vi "VoltageScan_datastream.vi"() -> ()   [LabVIEW 2015]
uses:
  Dynamic_data.ctl
  Program Files (x86)/National Instruments/LabVIEW 2016/instr.lib/Keithley 24XX/Keithley 24XX.lvlib
  Program Files (x86)/National Instruments/LabVIEW 2016/instr.lib/Agilent 428X Series/Agilent 428X Series.lvlib
  Program Files (x86)/National Instruments/LabVIEW 2016/instr.lib/Keithley 24XX/Public/Data/Read (Single Point).vi
  Input_parameters.ctl
panel:
  out "Voltages":cluster{"X":dbl[], "Y":dbl[]}[](graph) caption="XY Graph"
  out "Current channel":i32
  out "Channels":cluster{i32[], dbl[]}[](graph) caption="XY Graph"
  in  "Stop":bool
  out "Current voltage [V]":dbl
  out "Data curve for single channel":cluster{"X":dbl[], "Y":dbl[]}[](graph) caption="XY Graph"
  in  "Input parameters":T1={"Measurement type"=enum."Test", "Sensor type"=enum."One channel", "Input file"="", "Output file"="test.txt", "Open after execution?"=FALSE, "Display channel"=0, "Voltage Delay (s)"=0.5, "Switch Delay (s)"=0.01, "VISA resource name source"="", "VISA resource name LCR"="", "Voltage Limit (V)"=1000.0, "Enable Voltage Auto Range (T:Enable)"=TRUE, "Voltage Manual Range (1.0)"=1.0, "Compliance  Level (uA)"=10.0} {"Voltage Limit (V)" format="%#_13g"; "Voltage Delay (s)" format="%#_13g"; "Switch Delay (s)" format="%#_13g"}
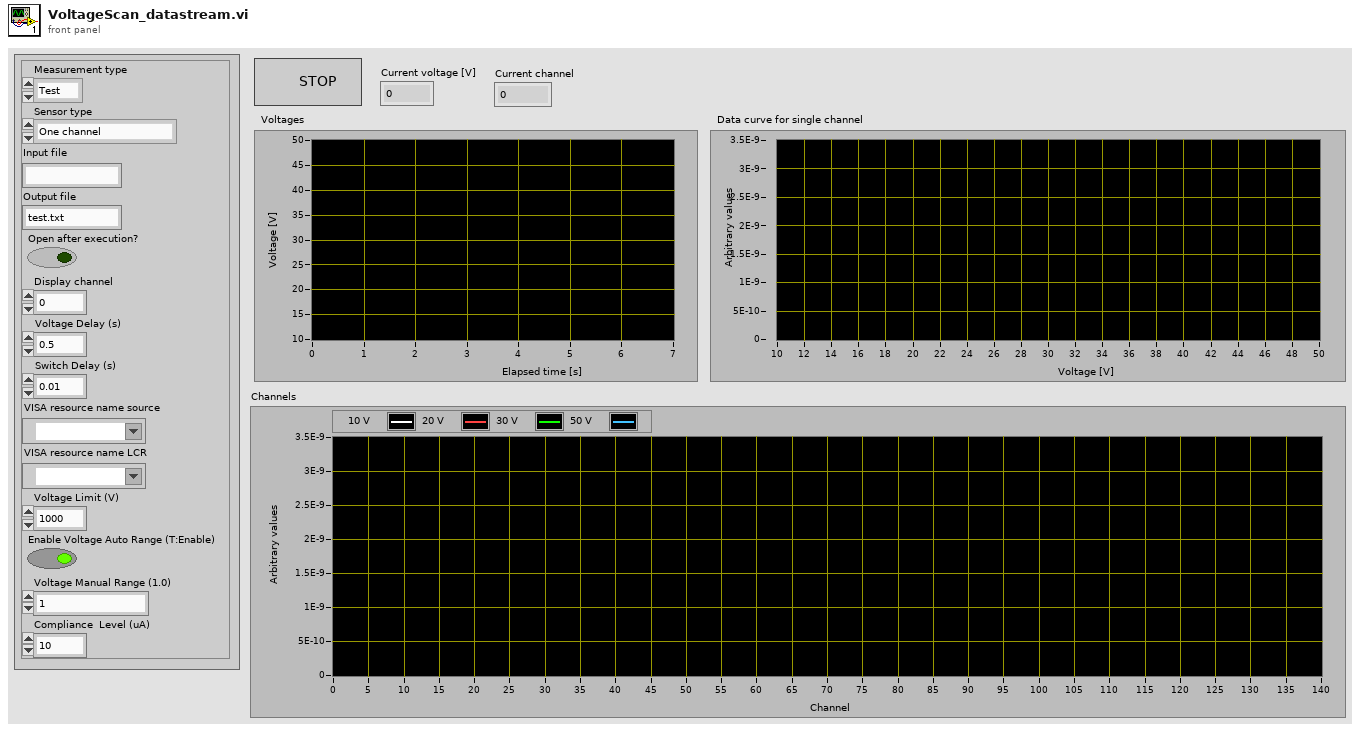
[diagram p1: front panel]
types:
  T1 = typedef "Input_parameters.ctl" = cluster{"Measurement type":enum16{"IV", "CV", "Test"}, "Sensor type":enum16{"6''", "8''", "One channel"}, "Input file":string, "Output file":string, "Open after execution?":bool, "Display channel":i32, "Voltage Delay (s)":dbl, "Switch Delay (s)":dbl, "VISA resource name source":refnum<visa-resource-name>, "VISA resource name LCR":refnum<visa-resource-name>, "Voltage Limit (V)":dbl, "Enable Voltage Auto Range (T:Enable)":bool, "Voltage Manual Range (1.0)":dbl, "Compliance  Level (uA)":dbl}
  T2 = typedef "Dynamic_data.ctl" = cluster{"Input file":path, "Output file":path, "Y-label text":string, "Voltage array":dbl[][], "Current set voltage":dbl, "Voltage column":dbl[], "Pad number column":dbl[], "Data  column":dbl[], "Number of voltages":i32, "Compliance current (A)":dbl}
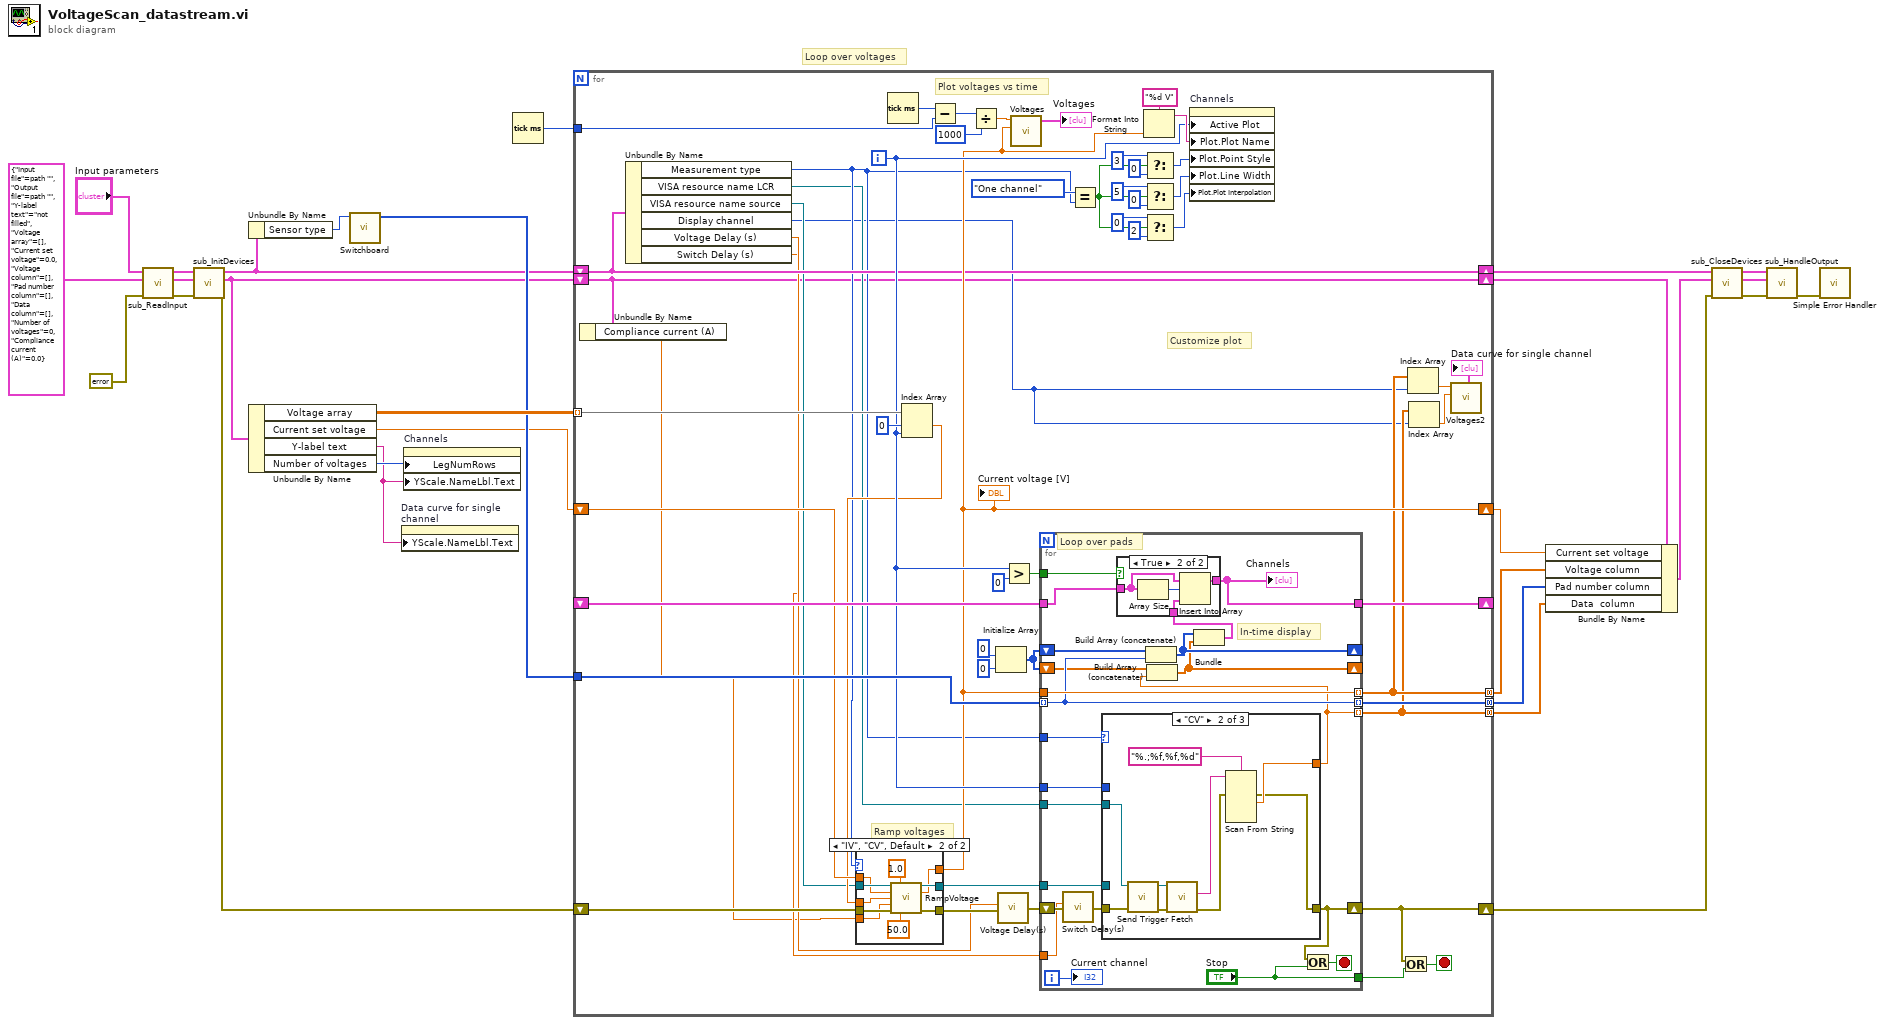
[diagram p0: block diagram]
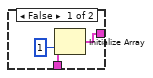
[diagram p3: hidden frame]
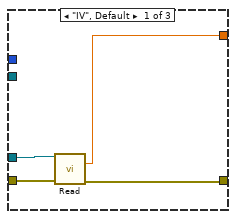
[diagram p4: hidden frame]
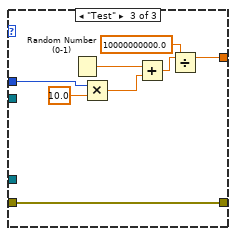
[diagram p5: hidden frame]
diagram:
  # "Loop over voltages"
  n1 = call "sub_ReadInput.vi"("error in (no error)"=errorcluster {"status"=FALSE, "code"=0, "source"=""}, "Dynamic data"=T2 {"Input file"=path "", "Output file"=path "", "Y-label text"="not filled", "Voltage array"=[], "Current set voltage"=0.0, "Voltage column"=[], "Pad number column"=[], "Data  column"=[], "Number of voltages"=0, "Compliance current (A)"=0.0}, "Input parameters"="Input parameters") -> ("error out"=w25:errorcluster, "Dynamic data"=w20:T2, "Input parameters"=w26:T1)  [unwired: 6 in]
  n2 = call "sub_InitDevices.vi"("error in (no error)"=w25, "Dynamic data"=w20, "Input parameters"=w26) -> ("error out"=w13:errorcluster, "Dynamic data"=w3:T2, "Input parameters"=w4:T1)  [unwired: 6 in]
  n3 = Unbundle By Name(w4) -> ("Sensor type"=w18:enum16{"6''", "8''", "One channel"})
  n4 = Unbundle By Name(w3) -> ("Voltage array"=w17:dbl[][], "Current set voltage"=w14:dbl, "Y-label text"=w5:string, "Number of voltages"=w6:i32)
  n5 = call "Switchboard.vi"("Sensor type"=w18) -> ("Output config"=w15:i32[])  [unwired: 10 in]
  n6 = property on="Data curve for single channel" class="XYGraph (strict)"("YScale.NameLbl.Text"=w5) -> ()  [unwired: 2 in, 2 out]
  n7 = property on="Channels" class="XYGraph (strict)"("LegNumRows"=w6, "YScale.NameLbl.Text"=w5) -> ()  [unwired: 2 in, 2 out]
  n8 = Tick Count (ms)() -> (millisecond timer value=w16:u32)
  n9 = for {
    tunnel: w17 -> [w83] mode=indexing
    tunnel: w15 -> [w80]
    tunnel: [w44] -> w9 mode=concatenating
    tunnel: [w43] -> w7 mode=concatenating
    tunnel: [w78] -> w8 mode=concatenating
    shift-right: [w48] -> w12
    shift-left: w13 -> [w76]
    shift-right: [w72] -> _
    shift-left: _ -> [w71]
    tunnel: w16 -> [w65]
    shift-right: [w45] -> w10
    shift-left: w14 -> [w47]
    shift-right: [w38] -> w2
    shift-left: w4 -> [w38]
    shift-right: [w30] -> w1
    shift-left: w3 -> [w30]
    i -> [w51]
    stop <- w49 stop-if-true
    # "Ramp voltages"
    # "Plot voltages vs time"
    # "Customize plot"
    n10 = Unbundle By Name(w30) -> ("Compliance current (A)"=w29:dbl)
    n11 = Unbundle By Name(w38) -> ("Measurement type"=w36:enum16{"IV", "CV", "Test"}, "VISA resource name LCR"=w34:refnum<visa-resource-name>, "VISA resource name source"=w35:refnum<visa-resource-name>, "Display channel"=w33:i32, "Voltage Delay (s)"=w32:dbl, "Switch Delay (s)"=w31:dbl)
    n12 = Tick Count (ms)() -> (millisecond timer value=w67:u32)
    n13 = Index Array(array=w83, index #1=0 ("index"), index #2=w51) -> (element #1=w46:dbl)  [unwired: 1 out]
    n14 = case shown="\"IV\", \"CV\", Default" w36 {
      tunnel: w35 -> [w86 w93]
      tunnel: w46 -> [w84 w92]
      tunnel: [w86 w95] -> w77
      tunnel: w76 -> [w85 w94]
      tunnel: [w85 w96] -> w75
      tunnel: w29 -> [_ w90]
      tunnel: w47 -> [_ w91]
      tunnel: [w84 w87] -> w45
      frame "Test" {
      }
      frame "IV", "CV", Default {
        n15 = call "RampVoltage.vi"("VISA resource name"=w93, "Delay (s)"=1.0, "Current voltage (V)"=w91, "Target voltage (V)"=w92, "Compliance Current (A)"=w90, "error in (no error)"=w94, "Step size (V)"=50.0) -> ("VISA resource name out"=w95:refnum<visa-resource-name>, "Current voltage out (V)"=w87:dbl, "error out"=w96:errorcluster)  [unwired: 6 in]
      }
    }
    "Current voltage [V]" <- w45
    n16 = Subtract(x=w67, y=w65) -> (x-y=w66:u32)
    n17 = Divide(x=w66, y=u32 1000 ("x")) -> (x/y=w64:dbl)
    n18 = Initialize Array(0 ("dimension size"), 0 ("dimension size")) -> (w68:i32[])
    n19 = call "Voltage Delay(s)"("error in (no error)"=w75, "Delay Time (s)"=w32) -> ("error out"=w74:errorcluster)  [unwired: 9 in]
    n20 = Greater?(x=w51, y=0) -> (0:w73:bool)
    n21 = call "Voltages"("Y Input"=w45, "X Input"=w64) -> ("XY Graph"=→"Voltages":cluster{"X":dbl[], "Y":dbl[]}[])  [unwired: 8 in, 1 out]
    n22 = for {
      tunnel: w80 -> [w114] mode=indexing
      tunnel: [w114] -> w78 mode=indexing
      tunnel: [w112] -> w43 mode=indexing
      tunnel: w45 -> [w118]
      tunnel: [w118] -> w44 mode=indexing
      tunnel: w77 -> [w116]
      tunnel: w36 -> [w117]
      shift-right: [w100] -> w48
      shift-left: w74 -> [w101]
      tunnel: w34 -> [w115]
      shift-right: [w110] -> _
      shift-left: w68 -> [w113]
      shift-right: [w109] -> _
      shift-left: w68 -> [w111]
      tunnel: w73 -> [w107]
      tunnel: w51 -> [w108]
      tunnel: w71 -> [w106]
      tunnel: [w104] -> w72
      tunnel: ["Stop"] -> w50
      tunnel: w31 -> [w97]
      i -> [w105]
      stop <- w99 stop-if-true
      # "In-time display"
      # "Loop over pads"
      n23 = call "Switch Delay(s)"("error in (no error)"=w101, "Delay Time (s)"=w97) -> ("error out"=w102:errorcluster)  [unwired: 9 in]
      n24 = case shown="\"CV\"" w117 {
        tunnel: [w129 w132 w140] -> w112
        tunnel: w116 -> [w127 _ _]
        tunnel: w102 -> [w128 w135 w146]
        tunnel: [w126 w130 w146] -> w100
        tunnel: w115 -> [_ w136 _]
        tunnel: w108 -> [_ _ w141]
        frame "IV", Default {
          n25 = call-poly "Read.vi"("VISA resource name"=w127, "error in (no error)"=w128) -> ("Current"=w129:sgl, "error out"=w126:errorcluster)  [unwired: 7 in, 5 out]
        }
        frame "CV" {
          n26 = call "Send Trigger.vi"("error in (no error)"=w135, "VISA resource name"=w136) -> ("error out"=w137:errorcluster, "VISA resource name out"=w138:refnum<visa-resource-name>)  [unwired: 8 in]
          n27 = call "Fetch.vi"("error in (no error)"=w137, "VISA resource name"=w138) -> ("error out"=w131:errorcluster, "Returned Data"=w133:string)  [unwired: 7 in, 1 out]
          n28 = Scan From String(format string="%.;%f,%f,%d", input string=w133, error in=w131) -> (error out=w130:errorcluster, output 1=w132:dbl)  [unwired: 6 in, 2 out]
        }
        frame "Test" {
          n29 = Random Number (0-1)() -> (number: 0 to 1=w145:dbl)
          n30 = Multiply(x=w141, y=10.0) -> (x*y=w142:dbl)
          n31 = Add(x=w145, y=w142) -> (x+y=w144:dbl)
          n32 = Divide(x=w144, y=10000000000.0) -> (x/y=w140:dbl)
        }
      }
      n33 = Build Array (concatenate)(w113, w114) -> (w110:i32[])
      n34 = Build Array (concatenate)(w111, w112) -> (w109:dbl[])
      n35 = Bundle(w110, w109) -> (w103:cluster{i32[], dbl[]})  [unwired: 1 out]
      n36 = case shown="True" w107 {
        tunnel: w106 -> [_ w124]
        tunnel: [w119 w123] -> w104
        tunnel: w103 -> [w120 w122]
        frame False {
          n37 = Initialize Array(w120, 1 ("dimension size")) -> (w119:cluster{i32[], dbl[]}[])
        }
        frame True {
          n38 = Array Size(array=w124) -> (size(s)=w125:i32)
          n39 = Insert Into Array(array=w124, index=w125, new element=w122) -> (w123:cluster{i32[], dbl[]}[])
        }
      }
      "Channels" <- w104
      n40 = Or(x=w100, y="Stop") -> (x .or. y?=w99:bool)
      "Current channel" <- w105
    }
    n41 = Equal?(x=enum16{"6''", "8''", "One channel"}."One channel" ("Sensor type 2"), y=w36) -> (x = y?=w37:bool)
    n42 = Format Into String(format string="%d V", w45) -> (resulting string=w62:string)  [unwired: 2 in, 1 out]
    n43 = Select(t=u8 3 ("Plot.Point Style"), s=w37, f=u8 0 ("Plot.Point Style")) -> (s? t:f=w57:u8)
    n44 = Select(t=u8 5 ("Plot.Point Style"), s=w37, f=u8 0 ("Plot.Point Style")) -> (s? t:f=w55:u8)
    n45 = Select(t=u8 0 ("Plot.Point Style"), s=w37, f=u8 2 ("Plot.Point Style")) -> (s? t:f=w52:u8)
    n46 = property on="Channels" class="XYGraph (strict)"("Active Plot"=w51, "Plot.Plot Name"=w62, "Plot.Point Style"=w57, "Plot.Line Width"=w55, "Plot.Plot Interpolation"=w52) -> ()  [unwired: 2 in, 2 out]
    n47 = Or(x=w48, y=w50) -> (x .or. y?=w49:bool)
    n48 = Index Array(array=w44, index=w33) -> (element=w41:dbl)
    n49 = Index Array(array=w43, index=w33) -> (element=w40:dbl)
    n50 = call "Voltages2"("Y Input"=w40, "X Input"=w41) -> ("XY Graph"=→"Data curve for single channel":cluster{"X":dbl[], "Y":dbl[]}[])  [unwired: 8 in, 1 out]
  }
  n51 = Bundle By Name(cluster=w1, "Current set voltage"=w10, "Voltage column"=w9, "Pad number column"=w8, "Data  column"=w7) -> (w11:T2)
  n52 = call "sub_CloseDevices.vi"("error in (no error)"=w12, "Dynamic data 2"=w11, "Input parameters"=w2) -> ("error out"=w24:errorcluster, "Dynamic data"=w19:T2, "Input parameters"=w23:T1)  [unwired: 6 in]
  n53 = call "sub_HandleOutput.vi"("error in (no error)"=w24, "Dynamic data 2"=w19, "Input parameters"=w23) -> ("error out"=w22:errorcluster)  [unwired: 6 in, 2 out]
  n54 = call <vilib>:"Simple Error Handler.vi"("error in (no error)"=w22) -> ()  [unwired: 4 in, 5 out]
